vi "Validate CONNECT.vi"(7 "JSON":string, 8 "error in":errorcluster, 11 "nats connection in":T1) -> (0 "error out":errorcluster, 2 "CONNECT msg":string, 3 "nats connection out":T1)   [LabVIEW 2013, in "NATS Core.lvlib"]
doc: "Uses a rudimentary approach to validate the JSON structure and creates the CONNECT message string"
uses:
  NATS Core.lvlib
  Controls/nats connection.ctl
  Package Version Constant.vi
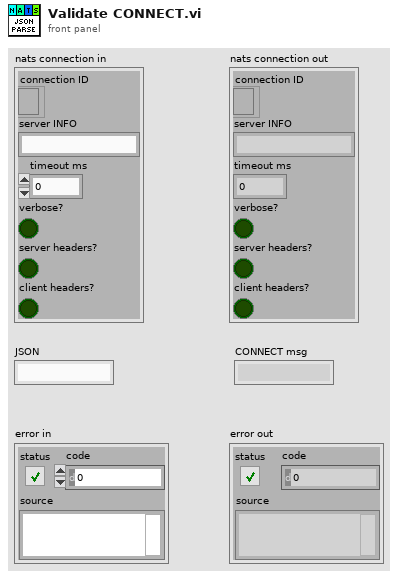
[diagram p1: front panel]
types:
  T1 = typedef "NATS Core.lvlib/nats connection.ctl" = cluster{"connection ID":refnum<k5>, "server INFO":string, "timeout ms":i32, "verbose?":bool, "server headers?":bool, "client headers?":bool}
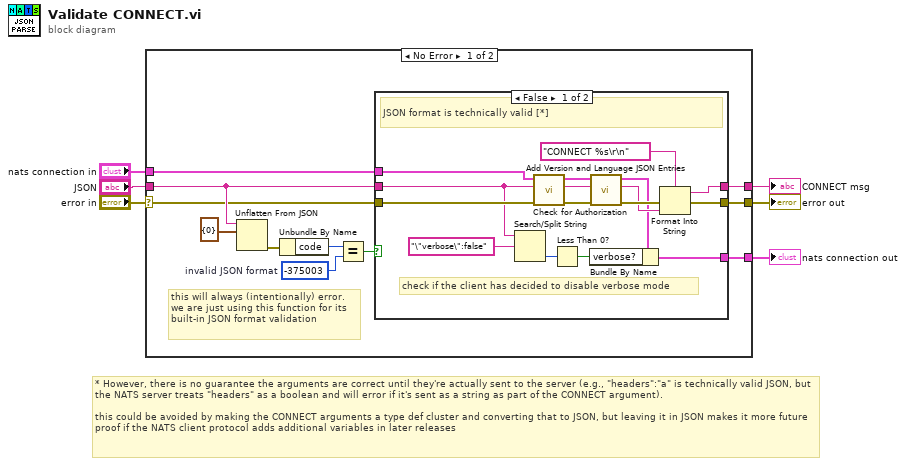
[diagram p0: block diagram]
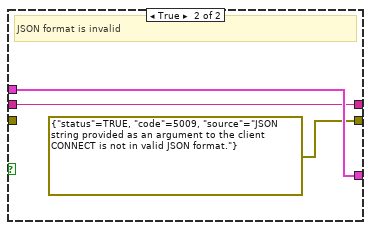
[diagram p2: hidden frame]
diagram:
  # "* However, there is no guarantee the arguments are correct until they're actually sent to the server (e.g., \"headers\":\"a\" is technically valid JSON, but the NATS server treats \"headers\" as a boolean and will error if it's sent as a string as part of the CONNECT argument).\n\nthis could be avoided by making the CONNECT arguments a type def cluster and converting that to JSON, but leaving it in JSON makes it more future proof if the NATS client protocol adds additional variables in later releases"
  n1 = case shown="No Error" "error in" {
    selector: "error in" -> [w13 w39]
    tunnel: "nats connection in" -> [w17 w38]
    tunnel: "JSON" -> [w16 w37]
    tunnel: [w14 w39] -> w3
    tunnel: [w12 w38] -> w2
    tunnel: [w11 w37] -> w1
    frame No Error {
      w8 = -375003  # invalid JSON format
      # "this will always (intentionally) error. we are just using this function for its built-in JSON format validation"
      n2 = Unflatten From JSON(JSON string=w16, type and defaults=cluster{i32} {0}) -> (error out=w10:errorcluster)  [unwired: 5 in, 1 out]
      n3 = Unbundle By Name(w10) -> ("code"=w9:i32)
      n4 = Equal?(x=w9, y=w8) -> (x = y?=w7:bool)
      n5 = case shown="False" w7 {
        tunnel: w17 -> [w20 w36]
        tunnel: w16 -> [w23 w35]
        tunnel: [w26 errorcluster {"status"=TRUE, "code"=5009, "source"="JSON string provided as an argument to the client CONNECT is not in valid JSON format."} ("error constant")] -> w14
        tunnel: w13 -> [w30 _]
        tunnel: [w29 w36] -> w12
        tunnel: [w24 w35] -> w11
        frame False {
          # "check if the client has decided to disable verbose mode"
          # "JSON format is technically valid [*]"
          n6 = Search/Split String(string=w23, search string/char (-)="\"verbose\":false") -> (offset of match=w31:i32)  [unwired: 1 in, 2 out]
          n7 = call "Check for Authorization.vi"("error in"=w30, "JSON"=w23, "nats connection in"=w20) -> ("error out"=w28:errorcluster, "dup JSON"=w21:string, "dup nats connection"=w22:T1)  [unwired: 6 in]
          n8 = Less Than 0?(x=w31) -> (x < 0?=w32:bool)
          n9 = call "Add Version and Language JSON Entries.vi"("error in"=w28, "JSON in"=w21, "nats connection in"=w22) -> ("error out"=w27:errorcluster, "JSON out"=w19:string, "nats connection out"=w18:T1)  [unwired: 6 in]
          n10 = Bundle By Name(cluster=w18, "verbose?"=w32) -> (w29:T1)
          n11 = Format Into String(format string="CONNECT %s\r\n", error in=w27, w19) -> (resulting string=w24:string, error out=w26:errorcluster)  [unwired: 1 in]
        }
        frame True {
          # "JSON format is invalid"
        }
      }
    }
    frame Error {
    }
  }
  "error out" <- w3
  "nats connection out" <- w2
  "CONNECT msg" <- w1
